vi "Acquire Datas.vi"(8 "error in (no error)":errorcluster, 11 "Acquire Data in":refnum<class "Acquire Data.lvclass">) -> (0 "error out":errorcluster, 1 "Currents":dbl[](array[numeric]), 2 "Volts":dbl[](array[numeric]), 3 "Acquire Data out":refnum<class "Acquire Data.lvclass">, 5 "Temps":dbl[](array[numeric]))   [LabVIEW 2018, in "Acquire Data.lvclass"]
uses:
  Acquire Data.lvclass
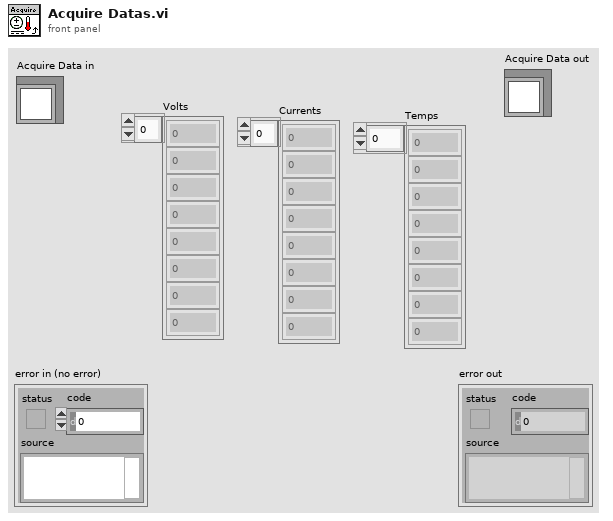
[diagram p1: front panel]
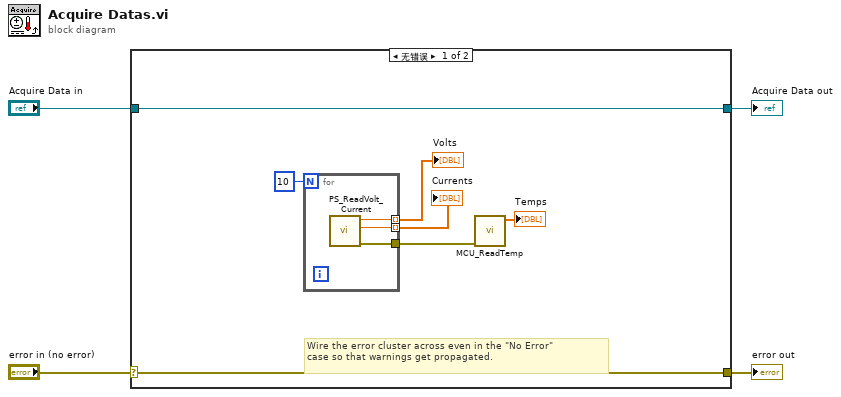
[diagram p0: block diagram]
diagram:
  n1 = case shown="无错误" "error in (no error)" {
    selector: "error in (no error)" -> [w10 w16]
    tunnel: [w10 w16] -> w3
    tunnel: [w11 w15] -> w1
    tunnel: "Acquire Data in" -> [w11 w15]
    frame No Error {
      # "Wire the error cluster across even in the \"No Error\"\ncase so that warnings get propagated."
      n2 = for {
        N: 10 -> [_]
        tunnel: [w13] -> w7 mode=indexing
        tunnel: [w14] -> w8
        tunnel: [w12] -> w6 mode=indexing
        n3 = call "PS_ReadVolt_Current.vi"() -> ("error out"=w14:errorcluster, "Current"=w12:dbl, "Volt"=w13:dbl)  [unwired: 9 in]
      }
      "Volts" <- w7
      "Currents" <- w6
      n4 = call "MCU_ReadTemp.vi"("error in (no error)"=w8) -> ("Volt"=→"Temps":dbl[])  [unwired: 9 in, 1 out]
    }
    frame Error {
    }
  }
  "error out" <- w3
  "Acquire Data out" <- w1
